vi "wave.vi"() -> (2 "sequenz":T1[](array[typedef]))   [LabVIEW 2022 SP3]
uses:
  angle_speed_def.ctl
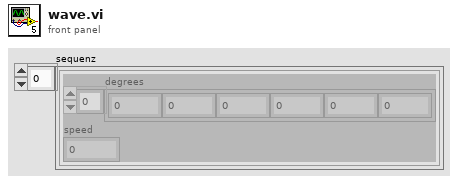
[diagram p1: front panel]
types:
  T1 = typedef "angle_speed_def.ctl" = cluster{"degrees":dbl[], "speed":i32}
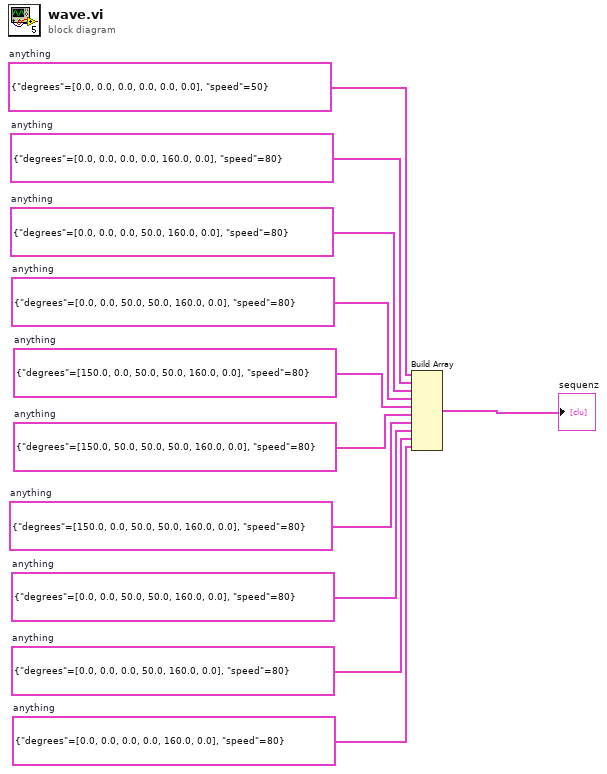
[diagram p0: block diagram]
diagram:
  w1 = T1 {"degrees"=[0.0, 0.0, 0.0, 0.0, 160.0, 0.0], "speed"=80}  # anything
  w3 = T1 {"degrees"=[0.0, 0.0, 50.0, 50.0, 160.0, 0.0], "speed"=80}  # anything
  w2 = T1 {"degrees"=[0.0, 0.0, 0.0, 50.0, 160.0, 0.0], "speed"=80}  # anything
  w4 = T1 {"degrees"=[150.0, 0.0, 50.0, 50.0, 160.0, 0.0], "speed"=80}  # anything
  w6 = T1 {"degrees"=[150.0, 0.0, 50.0, 50.0, 160.0, 0.0], "speed"=80}  # anything
  w5 = T1 {"degrees"=[150.0, 50.0, 50.0, 50.0, 160.0, 0.0], "speed"=80}  # anything
  w7 = T1 {"degrees"=[0.0, 0.0, 50.0, 50.0, 160.0, 0.0], "speed"=80}  # anything
  w9 = T1 {"degrees"=[0.0, 0.0, 0.0, 0.0, 160.0, 0.0], "speed"=80}  # anything
  w8 = T1 {"degrees"=[0.0, 0.0, 0.0, 50.0, 160.0, 0.0], "speed"=80}  # anything
  w10 = T1 {"degrees"=[0.0, 0.0, 0.0, 0.0, 0.0, 0.0], "speed"=50}  # anything
  n1 = Build Array(w10, w9, w8, w7, w6, w5, w4, w3, w2, w1) -> (→"sequenz":T1[])
